vi "Camera_Crop_Decluster.vi"(8 "input cluster":T1={"L16 Linear Actuator"="", "XE 1000 Pump"="", "Camera1"="", "Camera2"="", "Camera1_IMG"=refnum, "Camera2_IMG"=refnum, "Img_Capt"=FALSE, "Actuator"=FALSE, "Pump"=FALSE, "Cam 1"=FALSE, "Cam 2"=FALSE, "Empty_Refill"=FALSE, "Crop"=FALSE, "Light intensity"=100, "Exposure Time"=1000.0, "Sample Name"="Test Sample", "Operator"="MRJ", "Calibration 1"=path "C:/Users/au540322/Desktop/IHS_Project/images/Debris/Debris_0/Debris_0_2019_06_01-23-32-49-686.PNG", "Calibration 2"=path "C:/Users/au540322/Desktop/IHS_Project/images/Debris/Debris_0/Debris_0_2019_06_01-23-32-49-686.PNG", "Framerate"=100, "Timeout Sample"=200, "Collection date"="", "Sample size threshold"=500, "Empty start"=1, "Command"="", "Calibration Image 1"=refnum, "Calibration Image 2"=refnum, "Original Image 1"=refnum, "Original Image 2"=refnum, "Processing Image 1"=refnum, "Processing Image 2"=refnum, "Object Image 1"=refnum, "Object Image 2"=refnum, "Cam 1 - save queue"=refnum, "Cam 2 - save queue"=refnum, "Station"="", "Species Name"="", "Other Notes"="", "Aperture"=enum."Item 0", "Image Process Queue Size"=500, "Image Save Queue Size"=500, "Overload threshold"=500, "Max Framerate"=100, "Blue Plane Image"=refnum, "Subtract Image"=refnum, "Binary Image 1"=refnum, "ROI mask allocation"=refnum, "Rectangle 1"={"Left"=0, "Top"=0, "Right"=0, "Bottom"=0, "Rotation"=0.0}, "Rectangle 2"={"Left"=0, "Top"=0, "Right"=0, "Bottom"=0, "Rotation"=0.0}, "Binary Image 2"=refnum, "Detection Region %"=0.0, "Cam 1 queue"=refnum, "Cam 2 queue"=refnum, "Detect image 1"=refnum, "Detect image 2"=refnum, "Detect 1"=path "C:/Users/au540322/Desktop/IHS_Project/images/Debris/Debris_0/Debris_0_2019_06_01-23-32-49-686.PNG", "Detect 2"=path "C:/Users/au540322/Desktop/IHS_Project/images/Debris/Debris_0/Debris_0_2019_06_01-23-32-49-686.PNG", "Max large object threshold"=0, "Open(T)/Close(F)"=FALSE} {"Rectangle 2"."Rotation" format="%.2f"; "Rectangle 2"."Left" scale=0.0..1024.0; "Rectangle 2"."Right" scale=0.0..1024.0; "Rectangle 1"."Rotation" format="%.2f"; "Rectangle 1"."Left" scale=0.0..1024.0; "Rectangle 1"."Right" scale=0.0..1024.0; "Max Framerate" min=1; "Overload threshold" min=1; "Image Save Queue Size" min=1; "Image Process Queue Size" min=1; "Empty start" min=1; "Sample size threshold" min=1; "Framerate" min=1; "Light intensity" scale=0.0..100.0}, 10 "Detect Movement":bool, 11 "Camera":T5) -> (0 "OffsetY":i64, 1 "Height":i64, 2 "OffsetX":i64, 3 "Width":i64)   [LabVIEW 2019]
uses:
  Camera_ID.ctl
  controls/Data.ctl
  <vilib>/userdefined/High Color/IMAQdx.ctl
  <vilib>/vision/Image Controls.llb/IMAQ Image.ctl
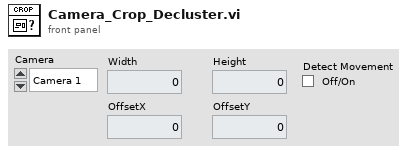
[diagram p1: front panel]
types:
  T1 = typedef "Data.ctl" = cluster{"L16 Linear Actuator":refnum<visa-resource-name>, "XE 1000 Pump":refnum<visa-resource-name>, "Camera1":T2, "Camera2":T2, "Camera1_IMG":T3, "Camera2_IMG":T3, "Img_Capt":bool, "Actuator":bool, "Pump":bool, "Cam 1":bool, "Cam 2":bool, "Empty_Refill":bool, "Crop":bool, "Light intensity":i32, "Exposure Time":dbl, "Sample Name":string, "Operator":string, "Calibration 1":path, "Calibration 2":path, "Framerate":i32, "Timeout Sample":i32, "Collection date":string, "Sample size threshold":i32, "Empty start":u32, "Command":string, "Calibration Image 1":T3, "Calibration Image 2":T3, "Original Image 1":T3, "Original Image 2":T3, "Processing Image 1":T3, "Processing Image 2":T3, "Object Image 1":T3, "Object Image 2":T3, "Cam 1 - save queue":refnum<queue>, "Cam 2 - save queue":refnum<queue>, "Station":string, "Species Name":string, "Other Notes":string, "Aperture":enum32{"Item 0", "Item 1", "Item 2", "Item 3"}, "Image Process Queue Size":i32, "Image Save Queue Size":i32, "Overload threshold":i32, "Max Framerate":i32, "Blue Plane Image":T3, "Subtract Image":T3, "Binary Image 1":T3, "ROI mask allocation":T3, "Rectangle 1":T4, "Rectangle 2":T4, "Binary Image 2":T3, "Detection Region %":dbl, "Cam 1 queue":refnum<queue>, "Cam 2 queue":refnum<queue>, "Detect image 1":T3, "Detect image 2":T3, "Detect 1":path, "Detect 2":path, "Max large object threshold":i32, "Open(T)/Close(F)":bool}
  T2 = typedef "IMAQdx.ctl" = refnum<k21>
  T3 = typedef "IMAQ Image.ctl" = refnum<image>
  T4 = typedef "IMAQ Rectangle" = cluster{"Left":i32, "Top":i32, "Right":i32, "Bottom":i32, "Rotation":dbl}
  T5 = typedef "Camera_ID.ctl" = enum16{"Camera 1", "Camera 2"}
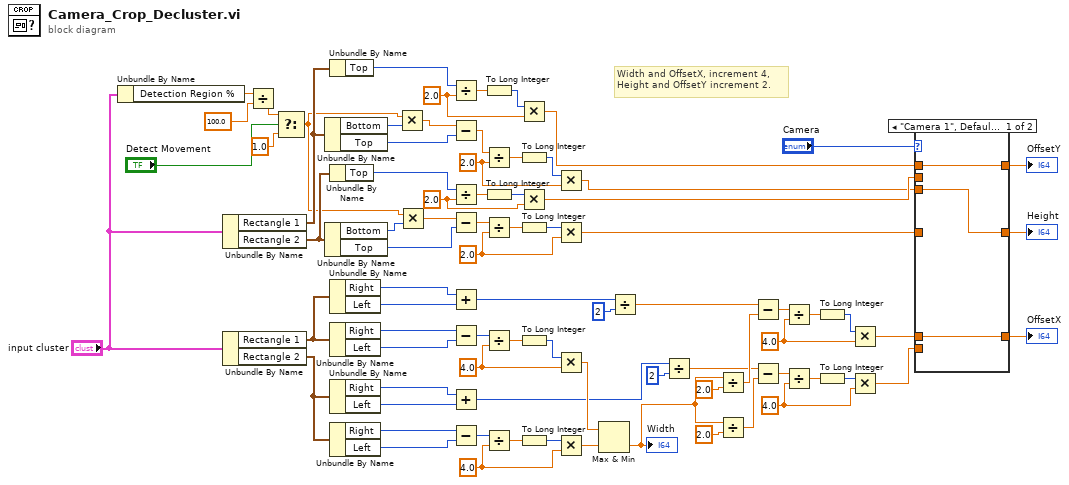
[diagram p0: block diagram]
diagram:
  w25 = 2.0 ("y")
  w28 = 2.0 ("y")
  w34 = 2.0 ("y")
  w13 = 2.0 ("y")
  w42 = 4.0 ("y")
  w46 = 4.0 ("y")
  w68 = 4.0 ("y")
  w73 = 4.0 ("y")
  # "Width and OffsetX, increment 4,\nHeight and OffsetY increment 2."
  n1 = Unbundle By Name("input cluster") -> ("Detection Region %"=w6:dbl)
  n2 = Unbundle By Name("input cluster") -> ("Rectangle 1"=w32:T4, "Rectangle 2"=w31:T4)
  n3 = Unbundle By Name("input cluster") -> ("Rectangle 1"=w64:T4, "Rectangle 2"=w51:T4)
  n4 = Divide(x=w6, y=100.0 ("x")) -> (x/y=w2:dbl)
  n5 = Select(t=w2, s="Detect Movement", f=1.0 ("t")) -> (s? t:f=w3:dbl)
  n6 = Unbundle By Name(w32) -> ("Bottom"=w11:i32, "Top"=w40:i32)
  n7 = Unbundle By Name(w31) -> ("Bottom"=w5:i32, "Top"=w39:i32)
  n8 = Unbundle By Name(w32) -> ("Top"=w16:i32)
  n9 = Unbundle By Name(w31) -> ("Top"=w15:i32)
  n10 = Unbundle By Name(w64) -> ("Right"=w63:i32, "Left"=w62:i32)
  n11 = Unbundle By Name(w64) -> ("Right"=w79:i32, "Left"=w78:i32)
  n12 = Unbundle By Name(w51) -> ("Right"=w55:i32, "Left"=w54:i32)
  n13 = Unbundle By Name(w51) -> ("Right"=w77:i32, "Left"=w76:i32)
  n14 = Multiply(x=w3, y=w11) -> (x*y=w10:dbl)
  n15 = Multiply(x=w3, y=w5) -> (x*y=w4:dbl)
  n16 = Divide(x=w16, y=w28) -> (x/y=w30:dbl)
  n17 = Subtract(x=w10, y=w40) -> (x-y=w37:dbl)
  n18 = Divide(x=w15, y=w25) -> (x/y=w27:dbl)
  n19 = Subtract(x=w4, y=w39) -> (x-y=w33:dbl)
  n20 = Add(x=w63, y=w62) -> (x+y=w61:i32)
  n21 = Subtract(x=w79, y=w78) -> (x-y=w72:i32)
  n22 = Add(x=w55, y=w54) -> (x+y=w53:i32)
  n23 = Subtract(x=w77, y=w76) -> (x-y=w67:i32)
  n24 = To Long Integer(number=w30) -> (32bit integer=w29:i32)
  n25 = Divide(x=w37, y=w13) -> (x/y=w38:dbl)
  n26 = To Long Integer(number=w27) -> (32bit integer=w26:i32)
  n27 = Divide(x=w33, y=w34) -> (x/y=w36:dbl)
  n28 = Divide(x=w72, y=w73) -> (x/y=w75:dbl)
  n29 = Divide(x=w67, y=w68) -> (x/y=w70:dbl)
  n30 = Multiply(x=w29, y=w28) -> (x*y=w22:dbl)
  n31 = To Long Integer(number=w38) -> (32bit integer=w14:i32)
  n32 = Multiply(x=w26, y=w25) -> (x*y=w19:dbl)
  n33 = To Long Integer(number=w36) -> (32bit integer=w35:i32)
  n34 = To Long Integer(number=w75) -> (32bit integer=w74:i32)
  n35 = To Long Integer(number=w70) -> (32bit integer=w69:i32)
  n36 = Multiply(x=w14, y=w13) -> (x*y=w12:dbl)
  n37 = Multiply(x=w35, y=w34) -> (x*y=w17:dbl)
  n38 = Multiply(x=w74, y=w73) -> (x*y=w71:dbl)
  n39 = Multiply(x=w69, y=w68) -> (x*y=w66:dbl)
  n40 = Max & Min(x=w71, y=w66) -> (min(x,y)=w49:dbl)  [unwired: 1 out]
  "Width" <- w49
  n41 = Divide(x=w61, y=2) -> (x/y=w59:dbl)
  n42 = Divide(x=w53, y=2) -> (x/y=w50:dbl)
  n43 = Divide(x=w49, y=2.0) -> (x/y=w58:dbl)
  n44 = Divide(x=w49, y=2.0) -> (x/y=w56:dbl)
  n45 = Subtract(x=w59, y=w58) -> (x-y=w45:dbl)
  n46 = Subtract(x=w50, y=w56) -> (x-y=w41:dbl)
  n47 = Divide(x=w45, y=w46) -> (x/y=w48:dbl)
  n48 = Divide(x=w41, y=w42) -> (x/y=w44:dbl)
  n49 = To Long Integer(number=w48) -> (32bit integer=w47:i32)
  n50 = To Long Integer(number=w44) -> (32bit integer=w43:i32)
  n51 = Multiply(x=w47, y=w46) -> (x*y=w24:dbl)
  n52 = Multiply(x=w43, y=w42) -> (x*y=w20:dbl)
  n53 = case shown="\"Camera 1\", Default" "Camera" {
    tunnel: w24 -> [w83 _]
    tunnel: [w83 w86] -> w23
    tunnel: w22 -> [w82 _]
    tunnel: [w82 w85] -> w21
    tunnel: w20 -> [_ w86]
    tunnel: w19 -> [_ w85]
    tunnel: [w81 w84] -> w18
    tunnel: w17 -> [_ w84]
    tunnel: w12 -> [w81 _]
    frame "Camera 1", Default {
    }
    frame "Camera 2" {
    }
  }
  "OffsetX" <- w23
  "OffsetY" <- w21
  "Height" <- w18
